vi "New Actor Message Transport.vi"(10 "Desired Notification Msg":refnum<class "Notification Msg.lvclass">) -> (0 "error out":errorcluster, 3 "ActorMessage out":refnum<class "ActorMessage.lvclass">)   [LabVIEW 2015, in "Mediator.lvlib" / "ActorMessage.lvclass"]
uses:
  ActorMessage.lvclass
  Transport Messages/Notification Msg/Notification Msg.lvclass
  ActorMessage.lvclass/ActorMessage.ctl
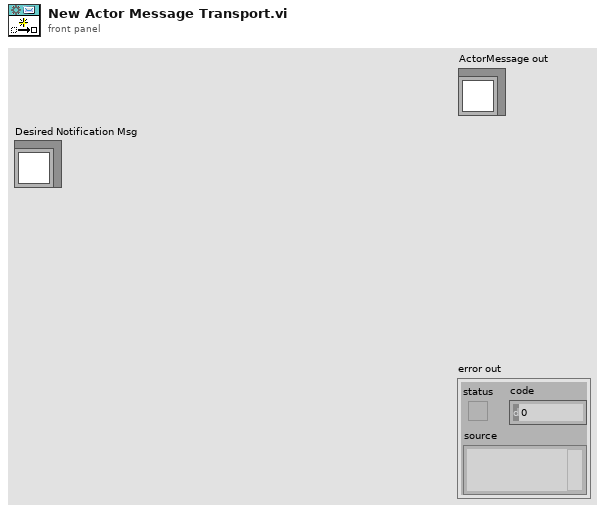
[diagram p1: front panel]
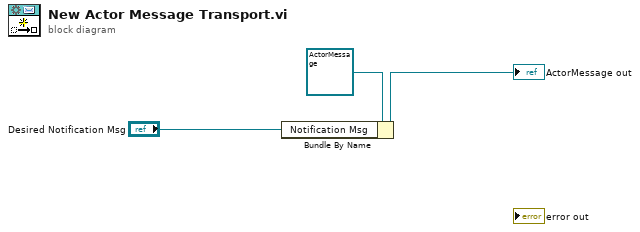
[diagram p0: block diagram]
diagram:
  n1 = Bundle By Name(cluster=refnum<class "ActorMessage.lvclass"> refnum ("ActorMessage in"), "Notification Msg"="Desired Notification Msg") -> (→"ActorMessage out":refnum<class "ActorMessage.lvclass">)
